vi "Sinal de PWM.vi"(2 "duty cycle":dbl(slide) scale=0.0..100.0, 3 "Frequência do PWM":dbl, 4 "Tempo atual":dbl) -> (0 "Resultado numérico":dbl, 1 "Resultado booleano":bool[](array[boolean]))   [LabVIEW 2018]
uses:
  <vilib>/express/express arith-compare/Formula/XNode/ExpressFormulaBlockNode.xnode
  <vilib>/gmath/NI_Gmath.lvlib
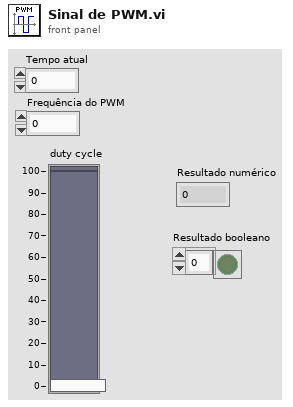
[diagram p1: front panel]
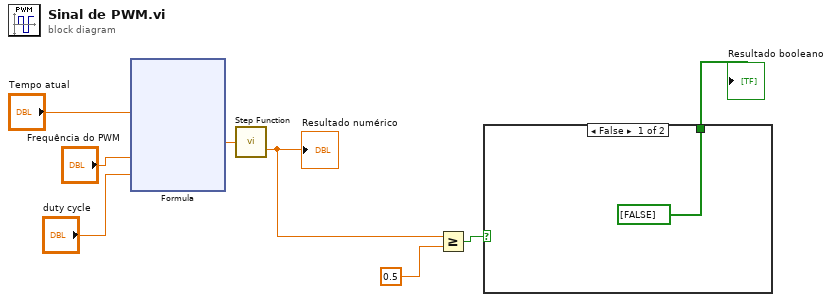
[diagram p0: block diagram]
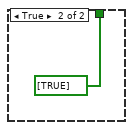
[diagram p2: hidden frame]
diagram:
  n1 = xnode "Formula"("t"="Tempo atual", "f"="Frequência do PWM", "dc"="duty cycle") -> ("Result"=w8:dbl)  [unwired: 1 in, 1 out]
  n2 = call <vilib>:"Step Function.vi"("x"=w8) -> ("step(x)"=w2:dbl)
  "Resultado numérico" <- w2
  n3 = Greater Or Equal?(x=w2, y=0.5) -> (x >= y?=w4:bool)
  n4 = case shown="False" w4 {
    tunnel: [bool[] [FALSE] ("data") bool[] [TRUE] ("data")] -> w3
    frame False {
    }
    frame True {
    }
  }
  "Resultado booleano" <- w3
